vi "Initialize Logger.vi"(8 "Error In":errorcluster, 11 "State Data":T1 {"Logging Data"."System Channel Refs" format="%.0x"; "Logging Data"."Block Data Refs"."Data Reference" format="%.0x"}) -> (0 "Error Out":errorcluster)   [LabVIEW 2019, in "Telemetry Engine.lvlib"]
uses:
  Telemetry Engine.lvlib
  Types/Engine State Data.ctl
  Types/Engine Logging Data.ctl
  <vilib>/NI VeriStand/Custom Device API/Custom Device Item Ref.ctl
  <vilib>/NI VeriStand/Custom Device API/Block Data Reference.ctl
  <vilib>/NI VeriStand/Custom Device API/Data Reference.ctl
  Types/Logger Data.ctl
  <vilib>/NI VeriStand/Custom Device API/Custom Device API.lvlib
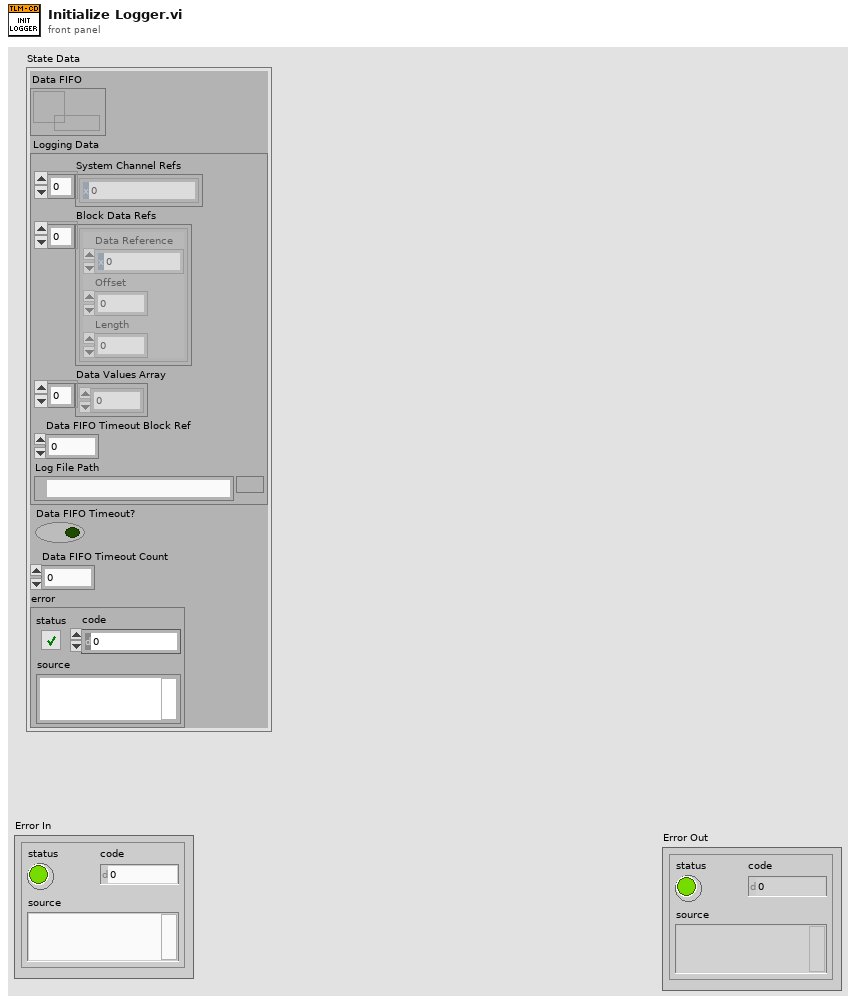
[diagram p1: front panel]
types:
  T1 = typedef "Telemetry Engine.lvlib/Engine State Data.ctl" = cluster{"Data FIFO":refnum<k33>, "Logging Data":T2, "Data FIFO Timeout?":bool, "Data FIFO Timeout Count":dbl, "error":errorcluster}
  T2 = typedef "Telemetry Engine.lvlib/Engine Logging Data.ctl" = cluster{"System Channel Refs":T3[], "Block Data Refs":T4[], "Data Values Array":dbl[], "Data FIFO Timeout Block Ref":i32, "Log File Path":path}
  T3 = typedef "Custom Device API.lvlib/Custom Device Item Ref.ctl" = u64
  T4 = typedef "Custom Device API.lvlib/Block Data Reference.ctl" = cluster{"Data Reference":T5, "Offset":u64, "Length":u64}
  T5 = typedef "Custom Device API.lvlib/Data Reference.ctl" = i32
  T6 = typedef "Telemetry Engine.lvlib/Logger Data.ctl" = cluster{"State":string, "Buffer size":i32, "Array Element size":i32, "Buffer Index":i32, "Data FIFO":refnum<k33>, "is Shutdown":bool, "Buffer":dbl[][], "Log path":path, "File ref":refnum<k34>, "Channel Names":string[], "Channel Descriptions":string[]}
  T7 = typedef "Custom Device API.lvlib/Custom Device Item Info.ctl" = cluster{"Name":string, "Is Channel":bool, "GUID":string, "Is Waveform":bool}
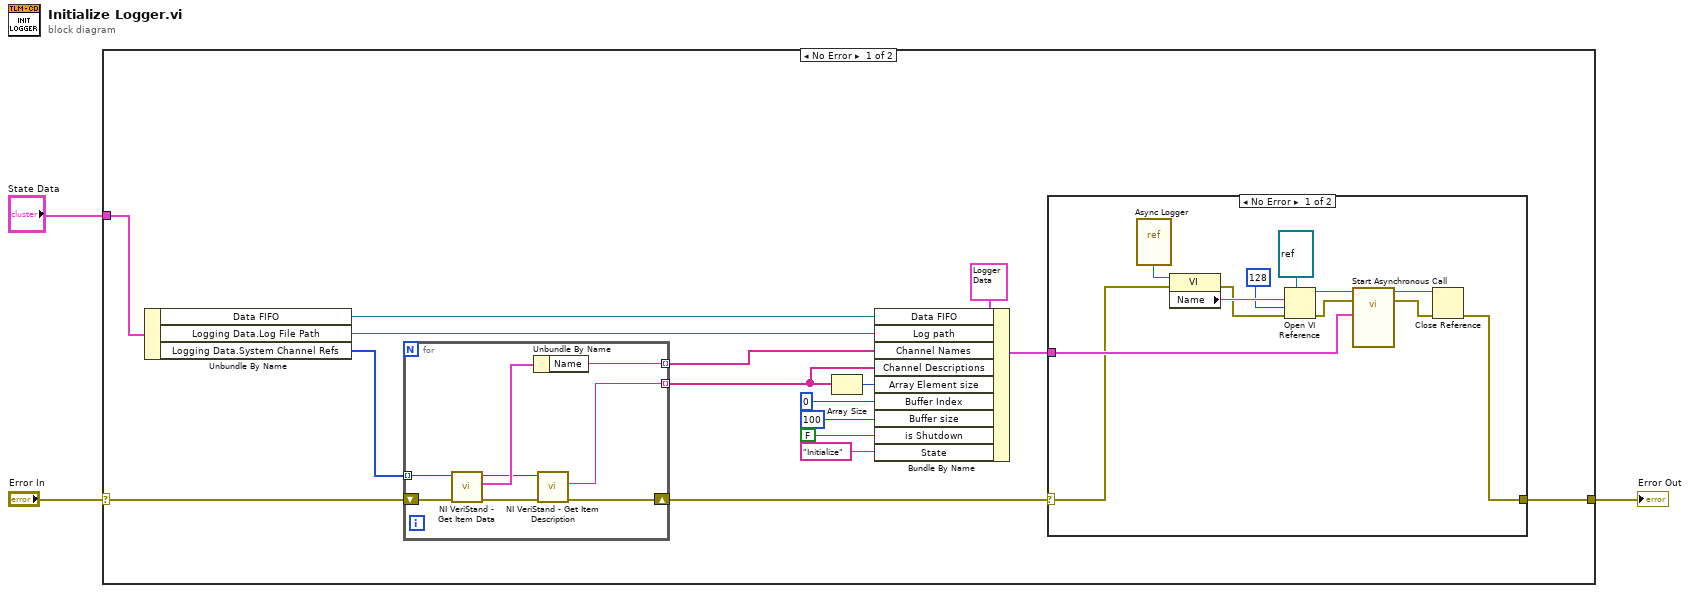
[diagram p0: block diagram]
diagram:
  n1 = case shown="No Error" "Error In" {
    selector: "Error In" -> [w17 w41]
    tunnel: "State Data" -> [w19 _]
    tunnel: [w8 w41] -> w1
    frame No Error {
      n2 = Unbundle By Name(w19) -> ("Data FIFO"=w11:refnum<k33>, "Logging Data.Log File Path"=w15:path, "Logging Data.System Channel Refs"=w18:T3[])
      n3 = for {
        tunnel: w18 -> [w38] mode=indexing
        shift-right: [w35] -> w7
        shift-left: w17 -> [w39]
        tunnel: [w34] -> w6 mode=indexing
        tunnel: [w33] -> w5 mode=indexing
        n4 = call <vilib>:"NI VeriStand - Get Item Data.vi"("error in (no error)"=w39, "Item Ref in"=w38) -> ("error out"=w36:errorcluster, "Item Info"=w40:T7, "Item Ref out"=w37:T3)  [unwired: 6 in, 1 out]
        n5 = Unbundle By Name(w40) -> ("Name"=w34:string)
        n6 = call <vilib>:"NI VeriStand - Get Item Description.vi"("error in (no error)"=w36, "Item Ref in"=w37) -> ("error out"=w35:errorcluster, "Description"=w33:string)  [unwired: 6 in, 2 out]
      }
      n7 = Array Size(array=w5) -> (size(s)=w4:i32)
      n8 = Bundle By Name(cluster=T6 {"State"="", "Buffer size"=0, "Array Element size"=0, "Buffer Index"=0, "Data FIFO"=refnum, "is Shutdown"=FALSE, "Buffer"=[], "Log path"=path "C:/logs/AdvancedTDMS_Telemetry_Prototype.tdms", "File ref"=refnum, "Channel Names"=[], "Channel Descriptions"=[]} ("Logger Parameters"), "Data FIFO"=w11, "Log path"=w15, "Channel Names"=w6, "Channel Descriptions"=w5, "Array Element size"=w4, "Buffer Index"=0, "Buffer size"=100, "is Shutdown"=FALSE, "State"="Initialize") -> (w9:T6)
      n9 = case shown="No Error" w7 {
        selector: w7 -> [w20 w32]
        tunnel: w9 -> [w22 _]
        tunnel: [w21 w32] -> w8
        frame No Error {
          n10 = vi-ref "Async Logger.vi"() -> (w27:refnum<vi>)
          n11 = property class="VI"(reference=w27, error in=w20) -> (error out=w25:errorcluster, "Name"=w26:string)  [unwired: 1 out]
          n12 = Open VI Reference(type specifier VI Refnum (for type only)=refnum<vi> refnum, vi path=w26, options=128 ("call and forget"), error in (no error)=w25) -> (vi reference=w31:refnum<vi>, error out=w30:errorcluster)  [unwired: 2 in]
          n13 = call-by-ref "Start Asynchronous Call"(reference=w31, error in=w30, "Logger Parameters"=w22) -> (reference out=w28:refnum<vi>, error out=w29:errorcluster)  [unwired: 9 in, 2 out]
          n14 = Close Reference(reference=w28, error in (no error)=w29) -> (error out=w21:errorcluster)
        }
        frame Error {
        }
      }
    }
    frame Error {
    }
  }
  "Error Out" <- w1
